vi "ADC Plot.vi"(3 "Channel 1":i32=105) -> ()   [LabVIEW 2015]
uses:
  Type/_RT Configuration 2.ctl
  Type/_RT Command.ctl
  <vilib>/printing/EasyPrintingControls.llb/layout_options.ctl
  <vilib>/printing/EasyPrintingControls.llb/orientation.ctl
  <vilib>/printing/EasyPrintingControls.llb/panel_scaling_for_page.ctl
  <vilib>/printing/EasyPrintingControls.llb/margins.ctl
  <vilib>/printing/EasyPrintingControls.llb/margin_values.ctl
  <vilib>/printing/EasyPrintingControls.llb/measurement_system.ctl
  <vilib>/printing/EasyPrintingControls.llb/printer_options.ctl
  <vilib>/printing/EasyPrintingControls.llb/printing_method.ctl
  <vilib>/printing/EasyPrintingControls.llb/color_or_monochrome.ctl
  <vilib>/printing/EasyPrintingControls.llb/page_header_options.ctl
  <vilib>/printing/EasyPrintingControls.llb/page_headers.ctl
  <vilib>/printing/EasyPrintingControls.llb/page_header_content_options.ctl
  <vilib>/printing/EasyPrinting.llb/Easy Print VI Panel or Documentation (path).vi
  <vilib>/Utility/NIReport.llb/NI_ReportGenerationCore.lvlib
panel:
  out "Name 6":string="Heater Current"
  in  "Channel 6":i32=14 caption="Channel 1"
  out "Name 5":string="P2T"
  in  "Channel 5":i32=108 caption="Channel 1"
  out "Name 4":string="HG2"
  in  "Channel 4":i32=68 caption="Channel 1"
  out "Name 3":string="P1T"
  in  "Channel 3":i32=110 caption="Channel 1"
  out "Name 2":string="HG1"
  in  "Channel 2":i32=67 caption="Channel 1"
  out "Start Time:":string
  out "Plot 1":cluster{dbl[], dbl[]}(graph) caption="Ch1 Plot"
  out "Plot 2":cluster{dbl[], dbl[]}(graph) caption="Ch1 Plot"
  out "Plot 3":cluster{dbl[], dbl[]}(graph) caption="Ch1 Plot"
  out "Plot 4":cluster{dbl[], dbl[]}(graph) caption="Ch1 Plot"
  out "Name 1":string="HSID T"
  in  "Start":bool
  out "Plot 6":cluster{dbl[], dbl[]}(graph) caption="Ch2 Plot"
  out "Plot 5":cluster{dbl[], dbl[]}(graph) caption="Ch1 Plot"
  in  "Stop":bool
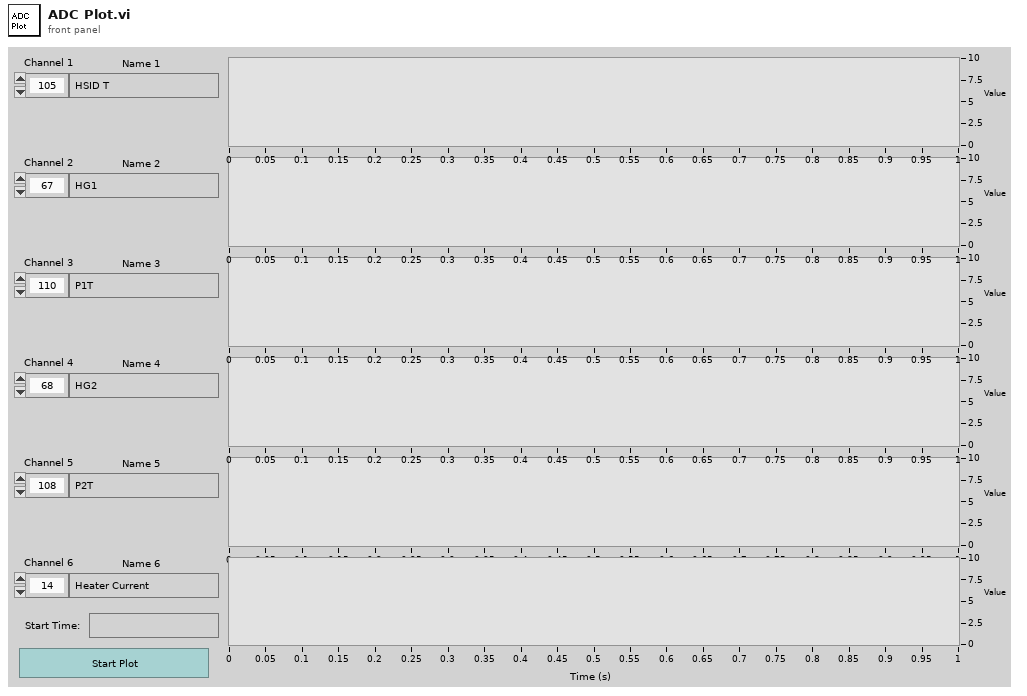
[diagram p1: front panel]
types:
  T1 = typedef "_RT Command.ctl" = enum16{"Start", "Stop", "Runtime Update", "Get Data", "Get Info", "Get Status", "Get Param", "Get Config", "Get Table", "Read ADC", "Set Oscillator", "Update Config", "Update Table", "Set All Pol", "Set Pol and DC", "Set Max Mass", "Toggle RP", "Toggle EL", "Set PIC", "Initialize Turbo", "Send Turbo Comm", "Close Turbo", "P1", "P2", "P3", "Send Serial", "Set LC Out", "Get LC In", "Read VAC", "Test Table", "Toggle Power", "Get Startup", "Set Startup", "Get ADC Table", "Set ADC Table", "Get Brief Status", "Get Detail Status", "Auxiliary Update", "Set CC Logics", "Set CC Input Logics", "Ignore Error"}
  T2 = typedef "NI_ReportGenerationCore.lvlib/layout_options.ctl" = cluster{"orientation (unchanged)":T3, "panel scaling for page (unchanged)":T4, "margins":T5, "printer options":T8, "page header options":T11}
  T3 = typedef "NI_ReportGenerationCore.lvlib/orientation.ctl" = u16
  T4 = typedef "NI_ReportGenerationCore.lvlib/panel_scaling_for_page.ctl" = u16
  T5 = typedef "NI_ReportGenerationCore.lvlib/margins.ctl" = cluster{"override VI margins (false)":bool, "margins (1.00)":T6, "measurement system (default)":T7}
  T6 = typedef "NI_ReportGenerationCore.lvlib/margin_values.ctl" = cluster{"top":dbl, "left":dbl, "right":dbl, "bottom":dbl}
  T7 = typedef "NI_ReportGenerationCore.lvlib/measurement_system.ctl" = u16
  T8 = typedef "NI_ReportGenerationCore.lvlib/printer_options.ctl" = cluster{"destination printer name (current)":string, "printing method (unchanged)":T9, "color or monochrome (unchanged)":T10}
  T9 = typedef "NI_ReportGenerationCore.lvlib/printing_method.ctl" = u16
  T10 = typedef "NI_ReportGenerationCore.lvlib/color_or_monochrome.ctl" = u16
  T11 = typedef "NI_ReportGenerationCore.lvlib/page_header_options.ctl" = cluster{"page headers (unchanged)":T12, "page header content options":T13}
  T12 = typedef "NI_ReportGenerationCore.lvlib/page_headers.ctl" = u16
  T13 = typedef "NI_ReportGenerationCore.lvlib/page_header_content_options.ctl" = cluster{"Include VI Name":bool, "Include VI Path":bool, "Include Last Modification Date":bool, "Include Date Printed":bool, "Include Page Number":bool, "Include VI Icon":bool}
  T14 = typedef "_RT Configuration 2.ctl" = cluster{"Name":string, "Ch#":u8, "Min":dbl, "Max":dbl, "Def+":dbl, "Def-":dbl, "Offset":dbl, "Slope":dbl, "Type":u8, "Description":string, "SettleT":dbl}
  T15 = typedef "imagedata.ctl" = cluster{"image type":i32, "image depth":i32, "image":u8[], "mask":u8[], "colors":u32[], "Rectangle":cluster{"left":i16, "top":i16, "right":i16, "bottom":i16}}
  T16 = enum8{"Enabled", "Disabled", "Disabled and Grayed Out"}
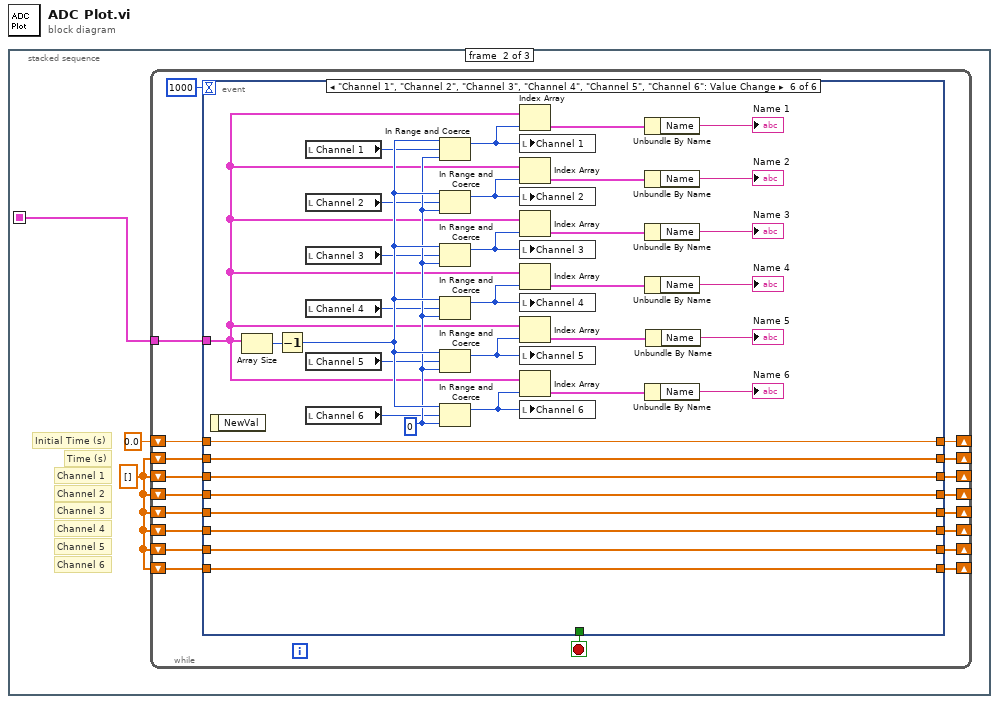
[diagram p0: block diagram]
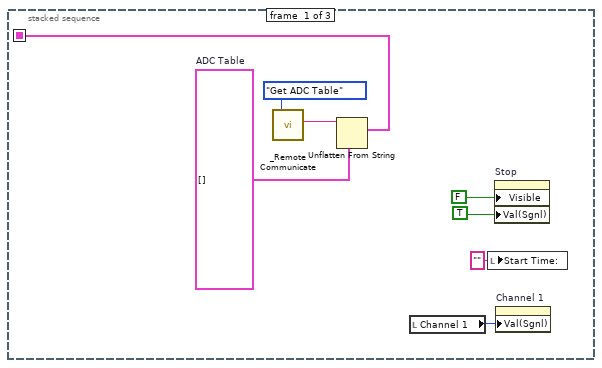
[diagram p2: hidden frame]
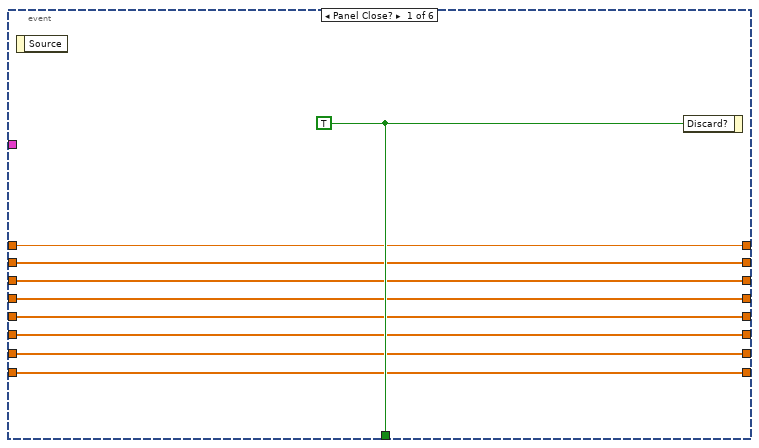
[diagram p3: hidden frame]
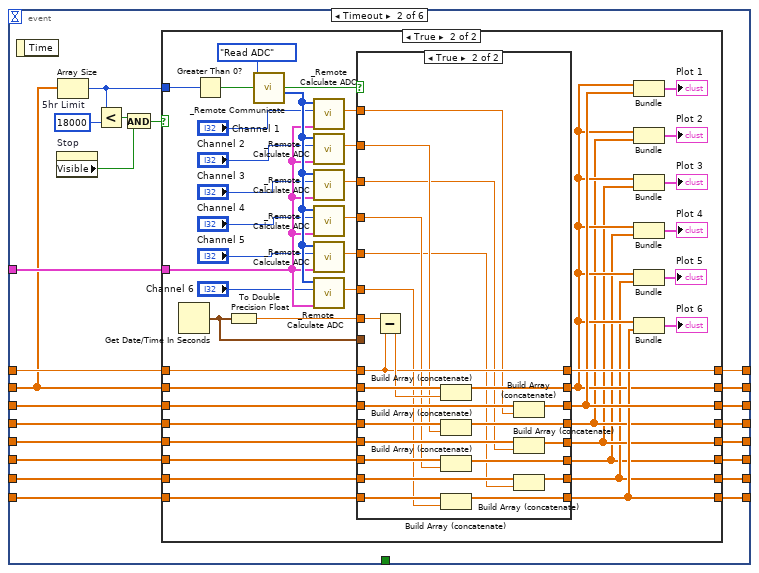
[diagram p4: hidden frame]
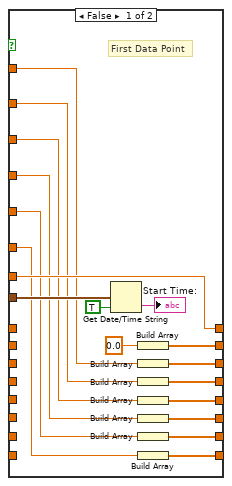
[diagram p6: hidden frame]
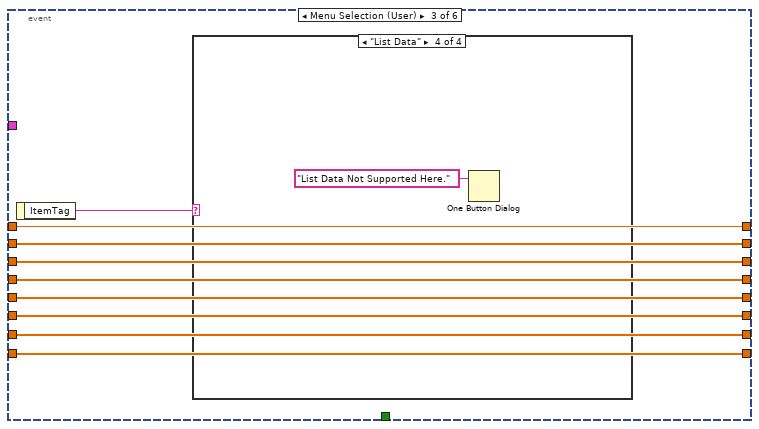
[diagram p7: hidden frame]
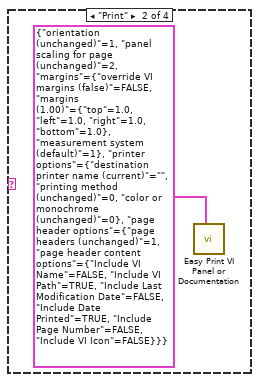
[diagram p9: hidden frame]
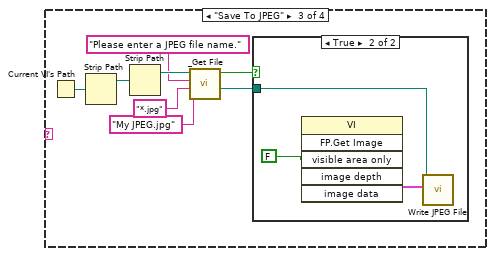
[diagram p10: hidden frame]
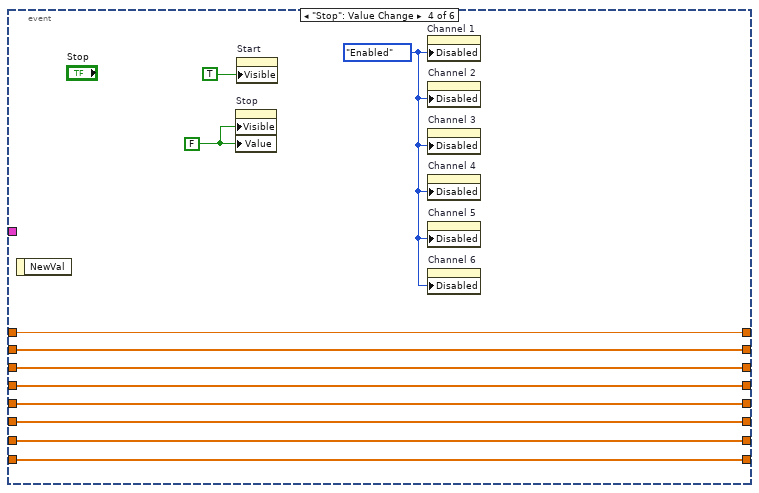
[diagram p12: hidden frame]
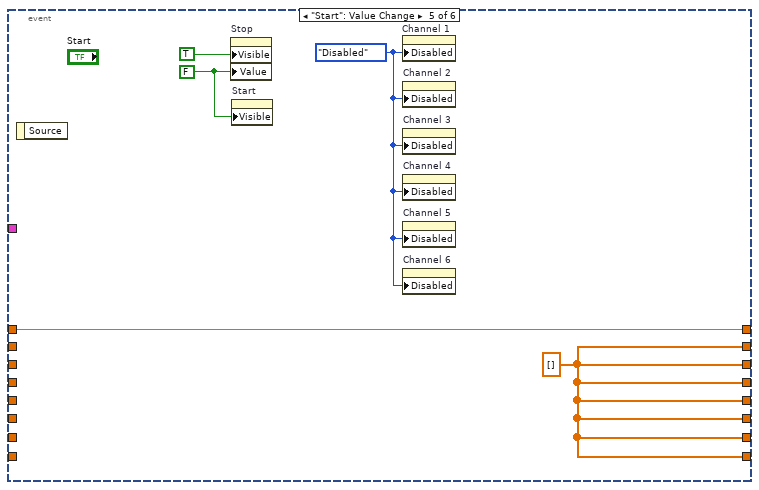
[diagram p13: hidden frame]
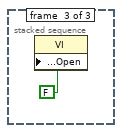
[diagram p14: hidden frame]
diagram:
  n1 = stacked-sequence {
    seq-local: [w2 _ _] -> [_ w11 _]
    frame #0 {
      w3 = T14[] []  # ADC Table
      n2 = call "_Remote Communicate.vi"("Command"=_RT_Command."Get ADC Table") -> ("Info"=w4:string)  [unwired: 5 in, 3 out]
      n3 = Unflatten From String(type=w3, binary string=w4) -> (value=w2:T14[])  [unwired: 1 in, 4 out]
      n4 = local read "Channel 1"() -> (w1:i32)
      n5 = local write "Start Time:"("" ("Start Time:")) -> ()
      n6 = property on="Stop" class="Bool (strict)"("Visible"=FALSE, "Val(Sgnl)"=TRUE ("Visible")) -> ()  [unwired: 2 in, 2 out]
      n7 = property on="Channel 1" class="DigNum (strict)"("Val(Sgnl)"=w1) -> ()  [unwired: 2 in, 2 out]
    }
    frame #1 {
      w9 = dbl[] []
      # "Initial Time (s)"
      # "Channel 6"
      # "Channel 5"
      # "Channel 4"
      # "Channel 3"
      # "Channel 2"
      # "Channel 1"
      # "Time (s)"
      n8 = while {
        shift-right: [w27] -> _
        shift-left: 0.0 -> [w28]
        tunnel: w11 -> [w26]
        shift-right: [w25] -> _
        shift-left: w9 -> [w23]
        shift-right: [w24] -> _
        shift-left: w9 -> [w22]
        shift-right: [w20] -> _
        shift-left: w9 -> [w21]
        shift-right: [w15] -> _
        shift-left: w9 -> [w19]
        shift-right: [w14] -> _
        shift-left: w9 -> [w18]
        shift-right: [w13] -> _
        shift-left: w9 -> [w17]
        shift-right: [w12] -> _
        shift-left: w9 -> [w16]
        stop <- w30 stop-if-true
        n9 = event shown="[5] \"Channel 1\", \"Channel 2\", \"Channel 3\", \"Channel 4\", \"Channel 5\", \"Channel 6\": Value Change" {
          selector: _ -> [_ _ _ _ _ _]
          dyn-events: _ -> [_ _ _ _ _ _]
          timeout: 1000 -> [_ _ _ _ _ _]
          tunnel: [w39 _ _ _ _ _] -> w30
          tunnel: w28 -> [w38 w56 w159 w182 w187 w224]
          tunnel: [w38 w55 w159 w182 w187 w224] -> w27
          tunnel: w26 -> [_ w54 _ _ _ w206]
          tunnel: [w37 w53 w158 w181 w185 w223] -> w25
          tunnel: [w36 w52 w157 w180 w185 w222] -> w24
          tunnel: w23 -> [w37 w49 w158 w181 _ w223]
          tunnel: w22 -> [w36 w57 w157 w180 _ w222]
          tunnel: w21 -> [w35 w50 w156 w179 _ w221]
          tunnel: [w35 w51 w156 w179 w185 w221] -> w20
          tunnel: [w34 w43 w155 w177 w185 w193] -> w15
          tunnel: w19 -> [w34 w47 w155 w177 _ w193]
          tunnel: [w33 w42 w154 w176 w185 w192] -> w14
          tunnel: w18 -> [w33 w46 w154 w176 _ w192]
          tunnel: [w32 w41 w153 w175 w185 w191] -> w13
          tunnel: w17 -> [w32 w45 w153 w175 _ w191]
          tunnel: [w31 w40 w152 w174 w185 w190] -> w12
          tunnel: w16 -> [w31 w44 w152 w174 _ w190]
          event Panel Close? {
            w39 = TRUE ("Discard?")
            n10 = event-data() -> ()  [unwired: 2 out]
            n11 = event-data("Discard?"=w39) -> ()  [unwired: 1 in, 1 out]
          }
          event Timeout {
            w61 = 18000  # 5hr Limit
            n12 = event-data() -> ()  [unwired: 2 out]
            n13 = property on="Stop" class="Bool (strict)"() -> ("Visible"=w59:bool)  [unwired: 2 in, 2 out]
            n14 = Array Size(array=w49) -> (size(s)=w48:i32)
            n15 = Less?(x=w48, y=w61) -> (x < y?=w60:bool)
            n16 = And(x=w60, y=w59) -> (x .and. y?=w58:bool)
            n17 = case shown="True" w58 {
              tunnel: w49 -> [w68 w107]
              tunnel: w57 -> [w67 w104]
              tunnel: w56 -> [w69 w106]
              tunnel: [w69 w105] -> w55
              tunnel: [w68 w78] -> w53
              tunnel: [w67 w82] -> w52
              tunnel: w54 -> [_ w93]
              tunnel: w50 -> [w66 w100]
              tunnel: [w66 w77] -> w51
              tunnel: w48 -> [_ w99]
              tunnel: w47 -> [w65 w98]
              tunnel: w46 -> [w64 w97]
              tunnel: w45 -> [w63 w96]
              tunnel: w44 -> [w62 w95]
              tunnel: [w65 w76] -> w43
              tunnel: [w64 w74] -> w42
              tunnel: [w63 w75] -> w41
              tunnel: [w62 w80] -> w40
              frame False {
              }
              frame True {
                n18 = Get Date/Time In Seconds() -> (seconds since 1Jan1904=w108:timestamp)
                n19 = Greater Than 0?(x=w99) -> (x > 0?=w110:bool)
                n20 = To Double Precision Float(number=w108) -> (double precision float=w109:dbl)
                n21 = call "_Remote Communicate.vi"("Command"=_RT_Command."Read ADC") -> ("Data Array"=w94:i32[])  [unwired: 5 in, 3 out]
                n22 = call "_Remote Calculate ADC.vi"("ADC Table"=w93, "ADC Channel (64)"="Channel 1", "ADC Values"=w94) -> ("User Value"=w89:dbl)  [unwired: 1 in, 3 out]
                n23 = call "_Remote Calculate ADC.vi"("ADC Table"=w93, "ADC Channel (64)"="Channel 2", "ADC Values"=w94) -> ("User Value"=w90:dbl)  [unwired: 1 in, 3 out]
                n24 = call "_Remote Calculate ADC.vi"("ADC Table"=w93, "ADC Channel (64)"="Channel 3", "ADC Values"=w94) -> ("User Value"=w91:dbl)  [unwired: 1 in, 3 out]
                n25 = call "_Remote Calculate ADC.vi"("ADC Table"=w93, "ADC Channel (64)"="Channel 4", "ADC Values"=w94) -> ("User Value"=w92:dbl)  [unwired: 1 in, 3 out]
                n26 = call "_Remote Calculate ADC.vi"("ADC Table"=w93, "ADC Channel (64)"="Channel 5", "ADC Values"=w94) -> ("User Value"=w101:dbl)  [unwired: 1 in, 3 out]
                n27 = call "_Remote Calculate ADC.vi"("ADC Table"=w93, "ADC Channel (64)"="Channel 6", "ADC Values"=w94) -> ("User Value"=w102:dbl)  [unwired: 1 in, 3 out]
                n28 = case shown="True" w110 {
                  tunnel: w109 -> [w124 w151]
                  tunnel: w108 -> [w126 _]
                  tunnel: w107 -> [_ w150]
                  tunnel: [w125 w148] -> w78
                  tunnel: w106 -> [_ w145]
                  tunnel: [w124 w145] -> w105
                  tunnel: w104 -> [_ w147]
                  tunnel: [w123 w146] -> w82
                  tunnel: w102 -> [w114 w129]
                  tunnel: w101 -> [w115 w130]
                  tunnel: w100 -> [_ w144]
                  tunnel: [w121 w143] -> w77
                  tunnel: w98 -> [_ w142]
                  tunnel: w97 -> [_ w141]
                  tunnel: w96 -> [_ w139]
                  tunnel: w95 -> [_ w140]
                  tunnel: w92 -> [w116 w131]
                  tunnel: w91 -> [w117 w132]
                  tunnel: w90 -> [w118 w133]
                  tunnel: w89 -> [w119 w134]
                  tunnel: [w120 w135] -> w80
                  tunnel: [w113 w138] -> w76
                  tunnel: [w112 w137] -> w74
                  tunnel: [w111 w136] -> w75
                  frame False {
                    # "First Data Point"
                    n29 = Get Date/Time String(seconds (now)=w126, want seconds? (F)=TRUE) -> (time string=→"Start Time:":string)  [unwired: 2 out]
                    n30 = Build Array(0.0) -> (w125:dbl[])
                    n31 = Build Array(w119) -> (w123:dbl[])
                    n32 = Build Array(w118) -> (w121:dbl[])
                    n33 = Build Array(w117) -> (w113:dbl[])
                    n34 = Build Array(w116) -> (w112:dbl[])
                    n35 = Build Array(w115) -> (w111:dbl[])
                    n36 = Build Array(w114) -> (w120:dbl[])
                  }
                  frame True {
                    n37 = Subtract(x=w151, y=w145) -> (x-y=w149:dbl)
                    n38 = Build Array (concatenate)(w150, w149) -> (w148:dbl[])
                    n39 = Build Array (concatenate)(w144, w133) -> (w143:dbl[])
                    n40 = Build Array (concatenate)(w141, w131) -> (w137:dbl[])
                    n41 = Build Array (concatenate)(w140, w129) -> (w135:dbl[])
                    n42 = Build Array (concatenate)(w147, w134) -> (w146:dbl[])
                    n43 = Build Array (concatenate)(w142, w132) -> (w138:dbl[])
                    n44 = Build Array (concatenate)(w139, w130) -> (w136:dbl[])
                  }
                }
                n45 = Bundle(w78, w82) -> (→"Plot 1":cluster{dbl[], dbl[]})  [unwired: 1 out]
                n46 = Bundle(w78, w77) -> (→"Plot 2":cluster{dbl[], dbl[]})  [unwired: 1 out]
                n47 = Bundle(w78, w76) -> (→"Plot 3":cluster{dbl[], dbl[]})  [unwired: 1 out]
                n48 = Bundle(w78, w74) -> (→"Plot 4":cluster{dbl[], dbl[]})  [unwired: 1 out]
                n49 = Bundle(w78, w75) -> (→"Plot 5":cluster{dbl[], dbl[]})  [unwired: 1 out]
                n50 = Bundle(w78, w80) -> (→"Plot 6":cluster{dbl[], dbl[]})  [unwired: 1 out]
              }
            }
          }
          event Menu Selection (User) {
            n51 = event-data() -> ("ItemTag"=w160:string)  [unwired: 1 out]
            n52 = case shown="\"List Data\"" w160 {
              frame Default {
              }
              frame "Print" {
                n53 = call-poly <vilib>:"Easy Print VI Panel or Documentation.vi"("layout options"=T2 {"orientation (unchanged)"=1, "panel scaling for page (unchanged)"=2, "margins"={"override VI margins (false)"=FALSE, "margins (1.00)"={"top"=1.0, "left"=1.0, "right"=1.0, "bottom"=1.0}, "measurement system (default)"=1}, "printer options"={"destination printer name (current)"="", "printing method (unchanged)"=0, "color or monochrome (unchanged)"=0}, "page header options"={"page headers (unchanged)"=1, "page header content options"={"Include VI Name"=FALSE, "Include VI Path"=TRUE, "Include Last Modification Date"=FALSE, "Include Date Printed"=TRUE, "Include Page Number"=FALSE, "Include VI Icon"=FALSE}}}) -> ()  [unwired: 4 in, 7 out]
              }
              frame "Save To JPEG" {
                n54 = Current VI's Path() -> (path=w169:path)
                n55 = Strip Path(path=w169) -> (stripped path=w168:path)  [unwired: 1 out]
                n56 = Strip Path(path=w168) -> (stripped path=w167:path)  [unwired: 1 out]
                n57 = call "_Get File.vi"("default name"="My JPEG.jpg", "extension (isd)"="*.jpg", "prompt"="Please enter a JPEG file name.", "Start Path"=w167) -> ("Seleted File"=w162:path, "Succeeded"=w163:bool)  [unwired: 2 in, 2 out]
                n58 = case shown="True" w163 {
                  tunnel: w162 -> [_ w170]
                  frame False {
                  }
                  frame True {
                    n59 = invoke class="VI" method="FP.Get Image"("visible area only"=FALSE ("Visible Area Only")) -> ("image data"=w171:T15)  [unwired: 5 in, 5 out]
                    n60 = call <vilib>:"Write JPEG File.vi"("image data"=w171, "path to JPEG file"=w170) -> ()  [unwired: 1 in, 9 out]
                  }
                }
              }
              frame "List Data" {
                n61 = One Button Dialog(message="List Data Not Supported Here.") -> ()  [unwired: 2 out]
              }
            }
          }
          event "Stop": Value Change {
            w178 = T16."Enabled" ("Disabled")
            w183 = FALSE ("Visible")
            n62 = event-data() -> ()  [unwired: 2 out]
            n63 = property on="Stop" class="Bool (strict)"("Visible"=w183, "Value"=w183) -> ()  [unwired: 2 in, 2 out]
            n64 = property on="Start" class="Bool"("Visible"=TRUE) -> ()  [unwired: 2 in, 2 out]
            n65 = property on="Channel 1" class="DigNum (strict)"("Disabled"=w178) -> ()  [unwired: 2 in, 2 out]
            n66 = property on="Channel 2" class="DigNum (strict)"("Disabled"=w178) -> ()  [unwired: 2 in, 2 out]
            n67 = property on="Channel 3" class="DigNum (strict)"("Disabled"=w178) -> ()  [unwired: 2 in, 2 out]
            n68 = property on="Channel 4" class="DigNum (strict)"("Disabled"=w178) -> ()  [unwired: 2 in, 2 out]
            n69 = property on="Channel 5" class="DigNum (strict)"("Disabled"=w178) -> ()  [unwired: 2 in, 2 out]
            n70 = property on="Channel 6" class="DigNum (strict)"("Disabled"=w178) -> ()  [unwired: 2 in, 2 out]
          }
          event "Start": Value Change {
            w186 = T16."Disabled" ("Disabled")
            w185 = dbl[] []
            w188 = FALSE ("Visible")
            n71 = event-data() -> ()  [unwired: 2 out]
            n72 = property on="Stop" class="Bool (strict)"("Visible"=TRUE, "Value"=w188) -> ()  [unwired: 2 in, 2 out]
            n73 = property on="Start" class="Bool"("Visible"=w188) -> ()  [unwired: 2 in, 2 out]
            n74 = property on="Channel 1" class="DigNum (strict)"("Disabled"=w186) -> ()  [unwired: 2 in, 2 out]
            n75 = property on="Channel 2" class="DigNum (strict)"("Disabled"=w186) -> ()  [unwired: 2 in, 2 out]
            n76 = property on="Channel 3" class="DigNum (strict)"("Disabled"=w186) -> ()  [unwired: 2 in, 2 out]
            n77 = property on="Channel 4" class="DigNum (strict)"("Disabled"=w186) -> ()  [unwired: 2 in, 2 out]
            n78 = property on="Channel 5" class="DigNum (strict)"("Disabled"=w186) -> ()  [unwired: 2 in, 2 out]
            n79 = property on="Channel 6" class="DigNum (strict)"("Disabled"=w186) -> ()  [unwired: 2 in, 2 out]
          }
          event "Channel 1", "Channel 2", "Channel 3", "Channel 4", "Channel 5", "Channel 6": Value Change {
            w218 = 0 ("lower limit")
            n80 = event-data() -> ()  [unwired: 2 out]
            n81 = Array Size(array=w206) -> (size(s)=w225:i32)
            n82 = Decrement(x=w225) -> (x-1=w219:i32)
            n83 = local read "Channel 1"() -> (w217:i32)
            n84 = local read "Channel 2"() -> (w215:i32)
            n85 = local read "Channel 3"() -> (w214:i32)
            n86 = local read "Channel 4"() -> (w213:i32)
            n87 = local read "Channel 5"() -> (w212:i32)
            n88 = local read "Channel 6"() -> (w216:i32)
            n89 = In Range and Coerce(upper limit=w219, x=w217, lower limit=w218) -> (coerced(x)=w205:i32)  [unwired: 1 out]
            n90 = In Range and Coerce(upper limit=w219, x=w215, lower limit=w218) -> (coerced(x)=w204:i32)  [unwired: 1 out]
            n91 = In Range and Coerce(upper limit=w219, x=w214, lower limit=w218) -> (coerced(x)=w203:i32)  [unwired: 1 out]
            n92 = In Range and Coerce(upper limit=w219, x=w213, lower limit=w218) -> (coerced(x)=w202:i32)  [unwired: 1 out]
            n93 = In Range and Coerce(upper limit=w219, x=w212, lower limit=w218) -> (coerced(x)=w201:i32)  [unwired: 1 out]
            n94 = In Range and Coerce(upper limit=w219, x=w216, lower limit=w218) -> (coerced(x)=w200:i32)  [unwired: 1 out]
            n95 = Index Array(array=w206, index=w205) -> (element=w220:T14)
            n96 = local write "Channel 1"(w205) -> ()
            n97 = Index Array(array=w206, index=w204) -> (element=w211:T14)
            n98 = local write "Channel 2"(w204) -> ()
            n99 = Index Array(array=w206, index=w203) -> (element=w210:T14)
            n100 = local write "Channel 3"(w203) -> ()
            n101 = Index Array(array=w206, index=w202) -> (element=w209:T14)
            n102 = local write "Channel 4"(w202) -> ()
            n103 = Index Array(array=w206, index=w201) -> (element=w208:T14)
            n104 = local write "Channel 5"(w201) -> ()
            n105 = Index Array(array=w206, index=w200) -> (element=w207:T14)
            n106 = local write "Channel 6"(w200) -> ()
            n107 = Unbundle By Name(w220) -> ("Name"=→"Name 1":string)
            n108 = Unbundle By Name(w211) -> ("Name"=→"Name 2":string)
            n109 = Unbundle By Name(w210) -> ("Name"=→"Name 3":string)
            n110 = Unbundle By Name(w209) -> ("Name"=→"Name 4":string)
            n111 = Unbundle By Name(w207) -> ("Name"=→"Name 6":string)
            n112 = Unbundle By Name(w208) -> ("Name"=→"Name 5":string)
          }
        }
      }
    }
    frame #2 {
      n113 = property class="VI"("Front Panel.Open"=FALSE ("Front Panel Window:Open")) -> ()  [unwired: 2 in, 2 out]
    }
  }
